vi "Start Recording.vi"(8 "error in (no error)":errorcluster, 10 "User Configuration":T1={"Start"=500000.0, "End"=2000000.0, "Duration"=40.0, "Filter time constant"=0.004, "Repeat (-1: forever)"=1, "Update rate"=0.004, "Data storage folder"=path "C:/Data"} {"Update rate" min=0.001 max=10.0 step=0.001 format="%#_6ps"; "Repeat (-1: forever)" format="%.0p"; "Filter time constant" format="%#_6ps"; "Duration" format="%#_6ps"; "End" format="%#_6pHz"; "Start" format="%#_6pHz"}, 11 "Spectrum Recorder in":refnum<class "Spectrum Recorder.lvclass">) -> (0 "error out":errorcluster, 3 "Spectrum Recorder out":refnum<class "Spectrum Recorder.lvclass">)   [LabVIEW 2016, in "Spectrum Recorder.lvclass"]
uses:
  Spectrum Recorder.lvclass
  Spectrum Recorder Configuration.ctl
  Spectrum Recorder.lvclass/Spectrum Recorder.ctl
  Red Pitaya/RP Core/RP Transceiver/Receiver format.ctl
  Red Pitaya/RP Core/RP Transceiver/RP Transceiver.lvclass/RP Transceiver.ctl
  Red Pitaya/RP Core/RP Instrument/RP Instrument.lvclass/RP Instrument.ctl
  Red Pitaya/RP Core/RP Transceiver/Write Receiver format.vi
  Red Pitaya/RP Core/RP Instrument/Write DDS delay.vi
  Red Pitaya/RP Core/RP Transceiver/RP Transceiver.lvclass
  C:/github/NHMFL_Core/Libraries/Red Pitaya/RP Core/RP Instrument/RP Instrument.lvclass
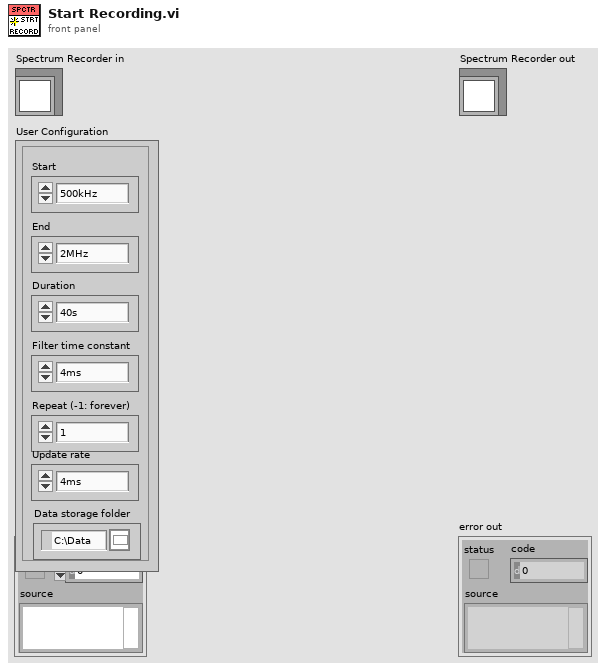
[diagram p1: front panel]
types:
  T1 = typedef "Spectrum Recorder Configuration.ctl" = cluster{"Start":dbl, "End":dbl, "Duration":dbl, "Filter time constant":dbl, "Repeat (-1: forever)":i32, "Update rate":dbl, "Data storage folder":path}
  T2 = typedef "Receiver format.ctl" = enum16{"X-Y-F", "F-X-Y", "X-Y", "X"}
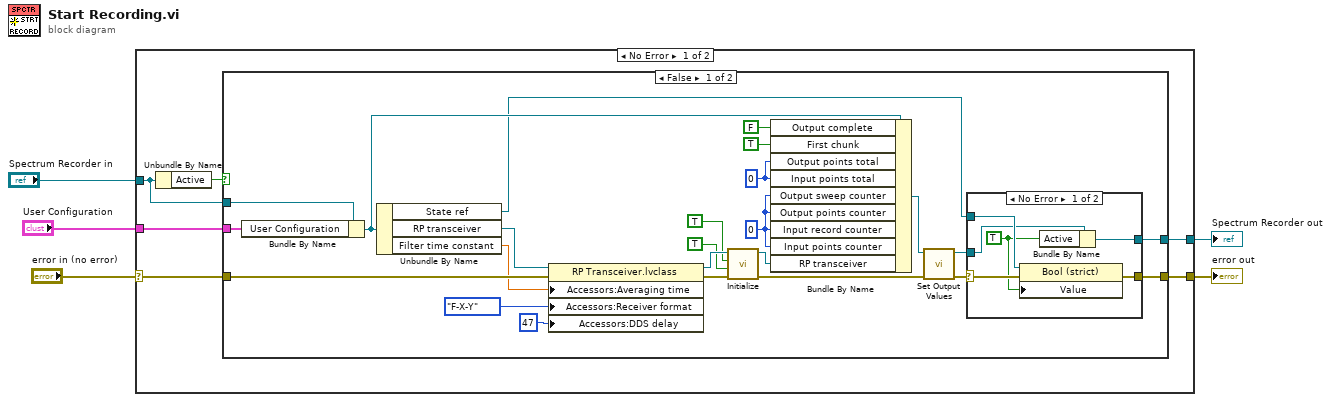
[diagram p0: block diagram]
diagram:
  n1 = case shown="No Error" "error in (no error)" {
    selector: "error in (no error)" -> [w7 w47]
    tunnel: [w6 w47] -> w4
    tunnel: [w11 w46] -> w2
    tunnel: "Spectrum Recorder in" -> [w9 w46]
    tunnel: "User Configuration" -> [w10 _]
    frame No Error {
      n2 = Unbundle By Name(w9) -> ("Active"=w8:bool)
      n3 = case shown="False" w8 {
        tunnel: w9 -> [w35 w45]
        tunnel: [w14 w45] -> w11
        tunnel: w10 -> [w34 _]
        tunnel: w7 -> [w30 w44]
        tunnel: [w21 w44] -> w6
        frame False {
          w13 = i64 0 ("Output points total")
          w19 = 0 ("Output sweep counter")
          n4 = Bundle By Name(cluster=w35, "User Configuration"=w34) -> (w33:refnum<class "Spectrum Recorder.lvclass">)
          n5 = Unbundle By Name(w33) -> ("State ref"=w20:refnum<vi>, "RP transceiver"=w23:refnum<class "RP Transceiver.lvclass">, "Filter time constant"=w24:dbl)
          n6 = property class="RP Transceiver.lvclass"(reference=w23, error in=w30, "Accessors:Averaging time"=w24, "Accessors:Receiver format"=Receiver_format."F-X-Y" ("Receiver format"), "Accessors:DDS delay"=u32 47 ("DDS delay")) -> (reference out=w29:refnum<class "RP Transceiver.lvclass">, error out=w28:errorcluster)
          n7 = call-dynamic "Initialize.vi"("error in (no error)"=w28, "Send \"Connect client\""=TRUE ("Send \"Connect client\""), "Reset"=TRUE, "RP Transceiver in"=w29) -> ("error out"=w25:errorcluster, "RP Transceiver out"=w17:refnum<class "RP Transceiver.lvclass">)  [unwired: 6 in]
          n8 = Bundle By Name(cluster=w33, "Output complete"=FALSE, "First chunk"=TRUE, "Output points total"=w13, "Input points total"=w13, "Output sweep counter"=w19, "Output points counter"=w19, "Input record counter"=w19, "Input points counter"=w19, "RP transceiver"=w17) -> (w22:refnum<class "Spectrum Recorder.lvclass">)
          n9 = call-dynamic "Set Output Values.vi"("error in (no error)"=w25, "Spectrum Recorder in"=w22) -> ("error out"=w16:errorcluster, "Spectrum Recorder out"=w15:refnum<class "Spectrum Recorder.lvclass">)  [unwired: 8 in]
          n10 = case shown="No Error" w16 {
            selector: w16 -> [w40 w42]
            tunnel: [w36 w42] -> w21
            tunnel: w20 -> [w41 _]
            tunnel: w15 -> [w39 w43]
            tunnel: [w38 w43] -> w14
            frame No Error {
              w37 = TRUE ("Value")
              n11 = property class="Bool (strict)"(reference=w41, error in=w40, "Value"=w37) -> (error out=w36:errorcluster)  [unwired: 1 out]
              n12 = Bundle By Name(cluster=w39, "Active"=w37) -> (w38:refnum<class "Spectrum Recorder.lvclass">)
            }
            frame Error {
            }
          }
        }
        frame True {
        }
      }
    }
    frame Error {
    }
  }
  "error out" <- w4
  "Spectrum Recorder out" <- w2
